vi "Stop DC meter.vi"(8 "error in (no error)":errorcluster, 11 "DC meter":T1={"DC meter type"=enum."H/A/K 3458", "DC meter VISA"="", "NPLC"=10.0}) -> (0 "error out":errorcluster, 3 "DC meter out":T1={"DC meter type"=enum."H/A/K 3458", "DC meter VISA"="", "NPLC"=10.0})   [LabVIEW 2020]
uses:
  Type definitions/DC meter.ctl
  Type definitions/DC meter type.ctl
  external libraries/Fluke 8508/Fluke 8508.lvlib
  external libraries/3458A Basic Driver/3458A Basic Driver.lvlib
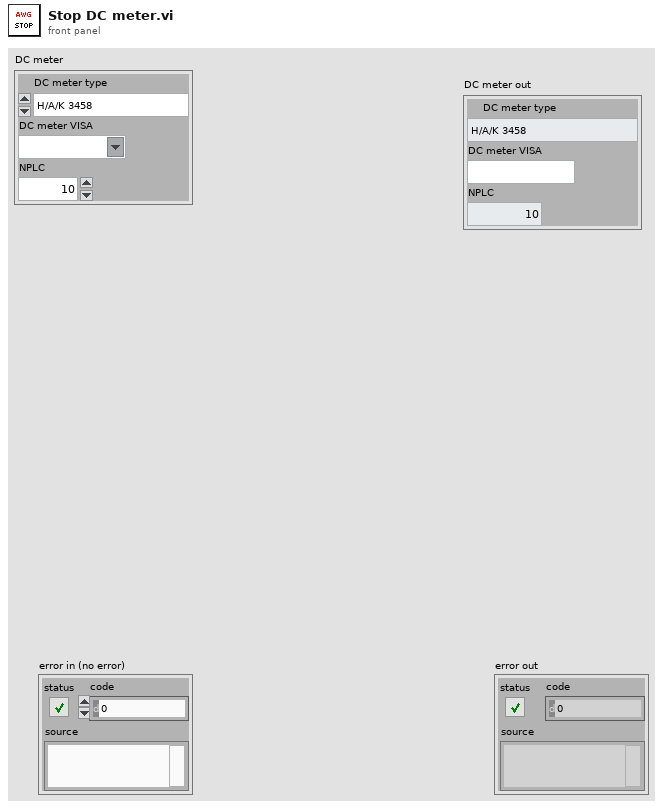
[diagram p1: front panel]
types:
  T1 = typedef "DC meter.ctl" = cluster{"DC meter type":T2, "DC meter VISA":refnum<visa-resource-name>, "NPLC":dbl}
  T2 = typedef "DC meter type.ctl" = enum16{"H/A/K 3458", "FLuke 8508A", "dummy"}
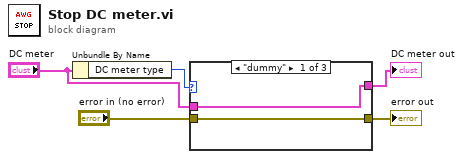
[diagram p0: block diagram]
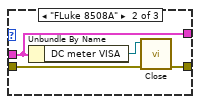
[diagram p2: hidden frame]
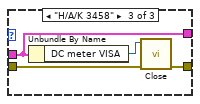
[diagram p3: hidden frame]
diagram:
  n1 = Unbundle By Name("DC meter") -> ("DC meter type"=w3:T2)
  n2 = case shown="\"dummy\"" w3 {
    tunnel: "error in (no error)" -> [w7 w9 w15]
    tunnel: [w7 w8 w14] -> w4
    tunnel: "DC meter" -> [w6 w11 w12]
    tunnel: [w6 w11 w12] -> w1
    frame "dummy" {
    }
    frame "FLuke 8508A" {
      n3 = Unbundle By Name(w11) -> ("DC meter VISA"=w10:refnum<visa-resource-name>)
      n4 = call "Close.vi"("error in (no error)"=w9, "VISA resource name"=w10) -> ("error out"=w8:errorcluster)  [unwired: 9 in]
    }
    frame "H/A/K 3458" {
      n5 = Unbundle By Name(w12) -> ("DC meter VISA"=w13:refnum<visa-resource-name>)
      n6 = call "Close.vi"("error in (no error)"=w15, "VISA resource name"=w13) -> ("error out"=w14:errorcluster)  [unwired: 9 in]
    }
  }
  "error out" <- w4
  "DC meter out" <- w1
